vi "Init.vi"(8 "error in (no error)":errorcluster, 11 "reference in":refnum<class "Test_Template.lvclass">) -> (0 "error out":errorcluster, 3 "reference out":refnum<class "Test_Template.lvclass">)   [LabVIEW 2019, in "Test_Template.lvlib" / "Test_Template.lvclass"]
uses:
  Test_Template.lvclass
  Components/Test_Base.lvlibp/Test_Base.lvclass
  Components/ViPER.lvlibp/ViPER.lvclass
  C:/Projects/Client-Nanosonics/Src/Components/ViPER.lvlibp/ViPER.lvclass
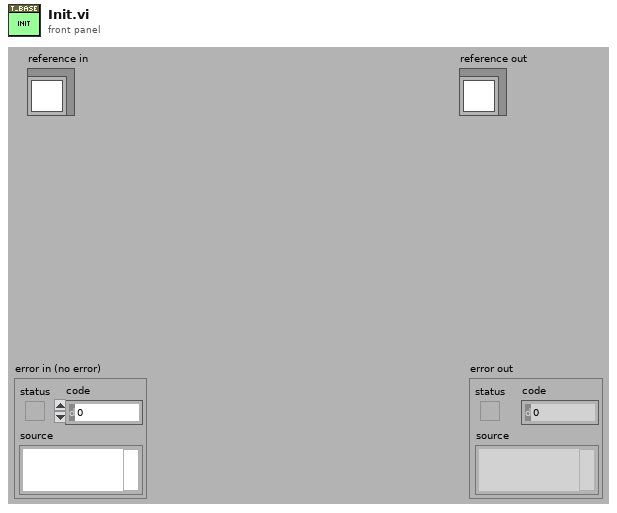
[diagram p1: front panel]
types:
  T1 = typedef "Test_Template.lvlib/Test_Template.lvclass/ObjectAttributes.ctl" = cluster{"Config":T2}
  T2 = typedef "Test_Template.lvlib/Test_Template.lvclass/Config.ctl" = cluster{"default":string}
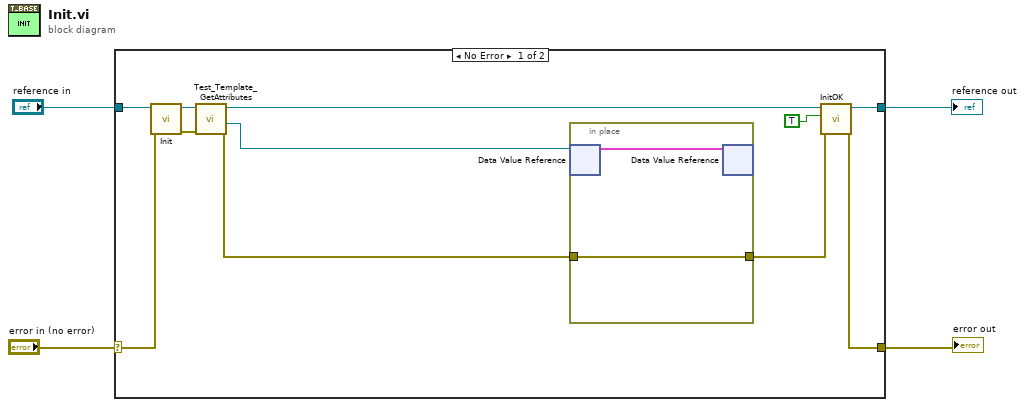
[diagram p0: block diagram]
diagram:
  n1 = case shown="No Error" "error in (no error)" {
    selector: "error in (no error)" -> [w14 w19]
    tunnel: [w7 w19] -> w3
    tunnel: [w10 w18] -> w1
    tunnel: "reference in" -> [w15 w18]
    frame No Error {
      n2 = call-parent "Init.vi"("error in (no error)"=w14, "reference in"=w15) -> ("error out"=w12:errorcluster, "reference out"=w13:refnum<class "Test_Template.lvclass">)  [unwired: 8 in]
      n3 = call "Test_Template_GetAttributes.vi"("error in (no error)"=w12, "reference in"=w13) -> ("error out"=w5:errorcluster, "DataRef"=w11:refnum<data-value>, "reference out"=w6:refnum<class "Test_Template.lvclass">)  [unwired: 6 in, 1 out]
      n4 = in-place {
        in-place-border: w5 -> [w17]
        in-place-border: [w17] -> w8
        n5 = in-place-dvr #1(w11) -> (w16:T1)  [unwired: 1 out]
        n6 = in-place-dvr #1(w16) -> ()  [unwired: 2 out]
      }
      n7 = call "InitOK.vi"("error in (no error)"=w8, "Init OK?"=TRUE, "reference in"=w6) -> ("error out"=w7:errorcluster, "reference out"=w10:refnum<class "Test_Template.lvclass">)  [unwired: 7 in]
    }
    frame Error {
    }
  }
  "error out" <- w3
  "reference out" <- w1
